vi "Object_Editor_SoftFP.vi"(0 "reference in":refnum<class "Object_Editor.lvclass">, 2 "Floating":bool, 5 "error in (no error)":errorcluster) -> (14 "reference out":refnum<class "Object_Editor.lvclass">, 19 "error out":errorcluster)   [LabVIEW 2022 SP3, in "Object_Editor.lvlib" / "Object_Editor.lvclass"]
uses:
  Object_Editor.lvclass
  <vilib>/picture/picture.llb/imagedata.ctl
  Components/ViPER.lvlibp/ViPER.lvclass
  C:/Projects/Medulla/ViPER/ViPER_ProjectTemplates/ProjectTemplates/Source/Core/ViPER/Components/ViPER.lvlibp/ViPER.lvclass
panel:
  in  "Object Tree":string(tree)
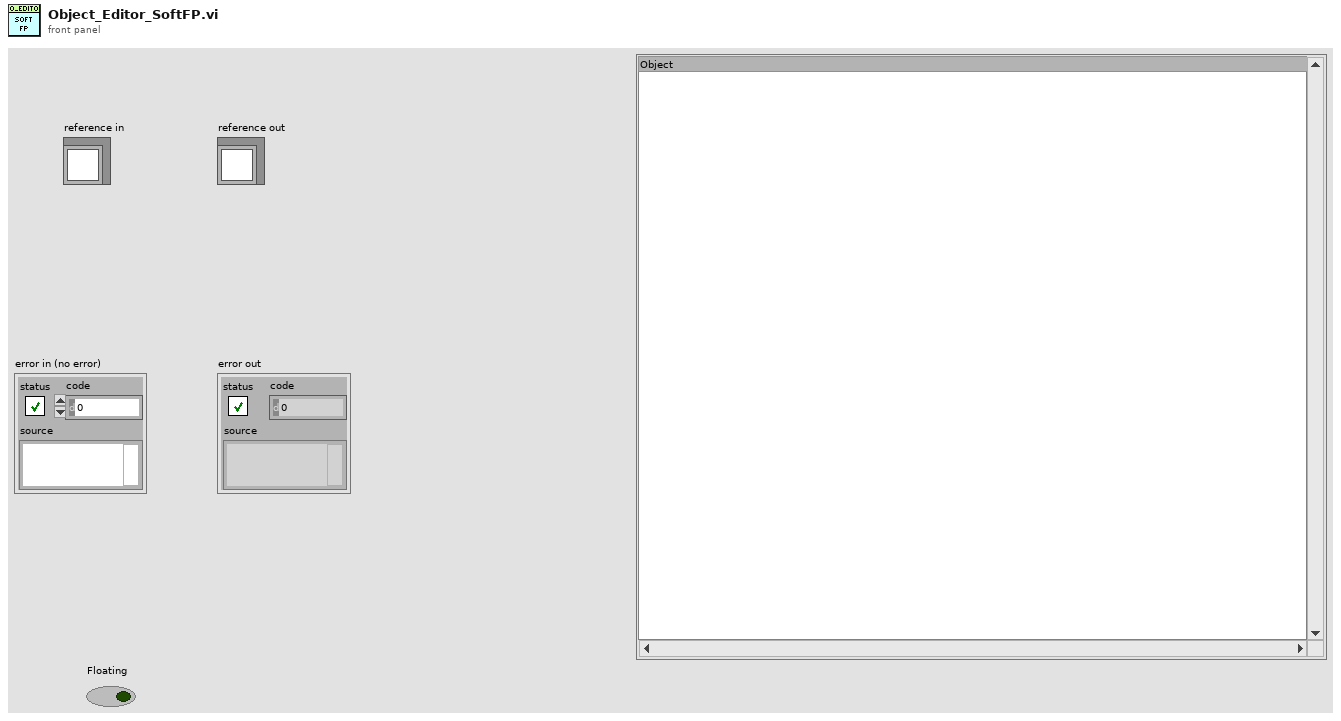
[diagram p1: front panel]
types:
  T1 = enum32{"Invalid", "Standard", "Closed", "Hidden", "Minimized", "Maximized"}
  T2 = typedef "imagedata.ctl" = cluster{"image type":i32, "image depth":i32, "image":u8[], "mask":u8[], "colors":u32[], "Rectangle":cluster{"left":i16, "top":i16, "right":i16, "bottom":i16}}
  T3 = typedef "Object_Editor.lvlib/Object_Editor.lvclass/ObjectAttributes.ctl" = cluster{"Config":T4, "Tree":refnum<vi>, "Mod_Bit":bool, "File_Path":path, "Object":refnum<class "ViPER.lvclass">}
  T4 = typedef "Object_Editor.lvlib/Object_Editor.lvclass/Config.ctl" = cluster{"default":string}
  T5 = typedef "LVPoint32TypeDef.ctl" = cluster{"Horizontal":i32, "Vertical":i32}
  T6 = typedef "Object_Editor.lvlib/Object_Editor.lvclass/TreeItem.ctl" = cluster{"Name":string, "Parent_Tag":string, "Child_Tag":string, "Type":T7, "Data":string}
  T7 = typedef "Object_Editor.lvlib/Object_Editor.lvclass/ItemType.ctl" = enum16{"Object", "Ancestor"}
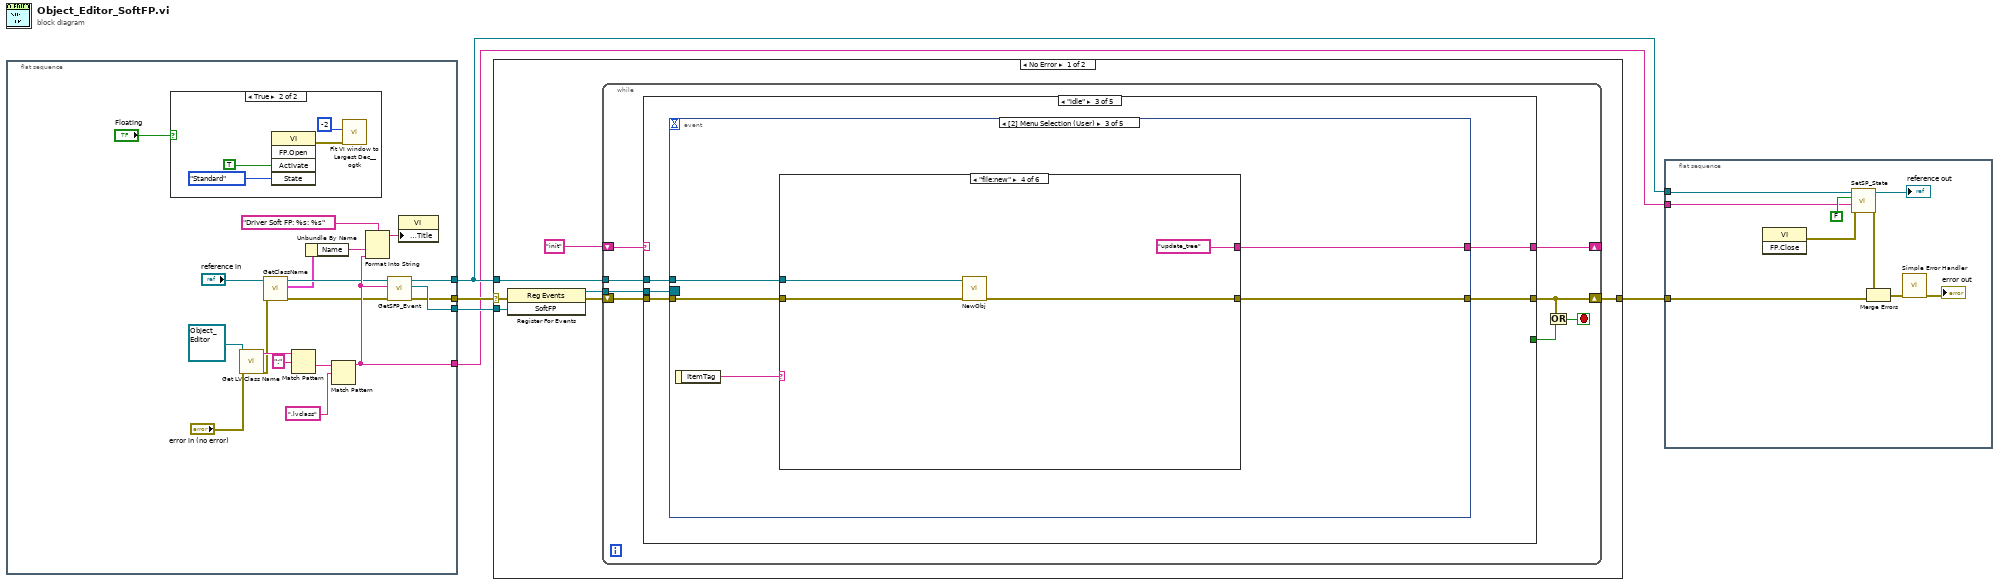
[diagram p0: block diagram]
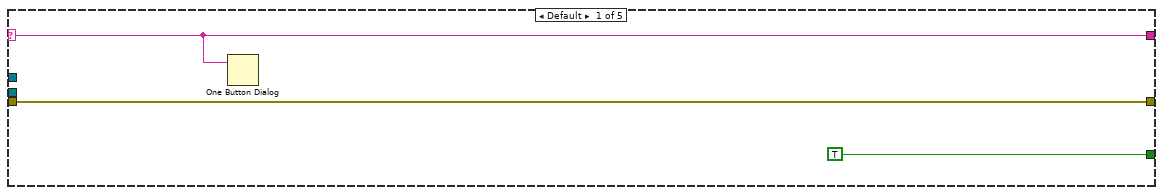
[diagram p3: hidden frame]
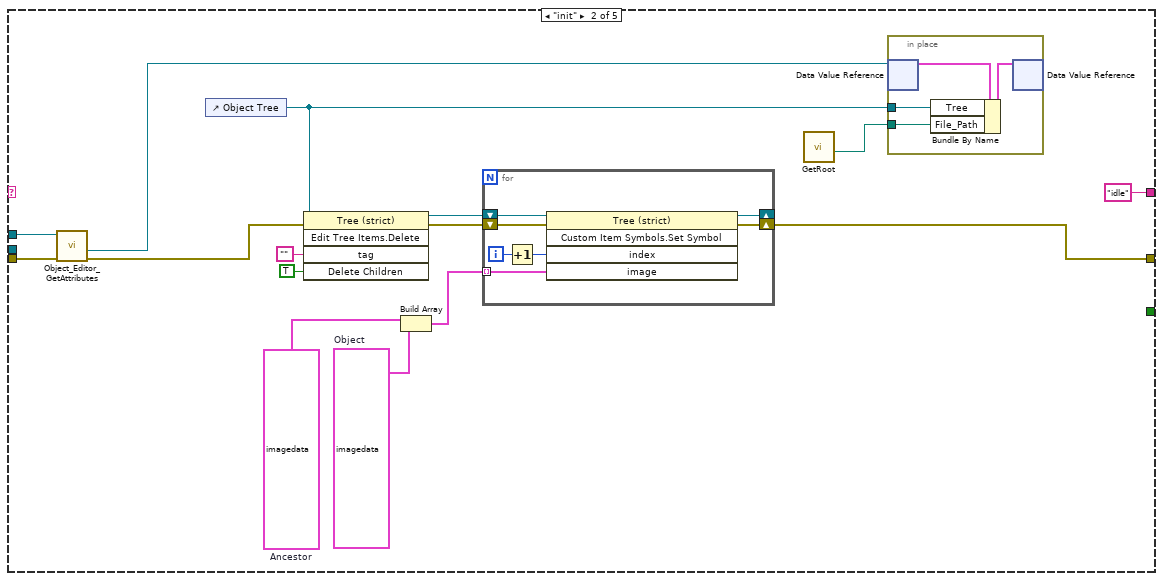
[diagram p4: hidden frame]
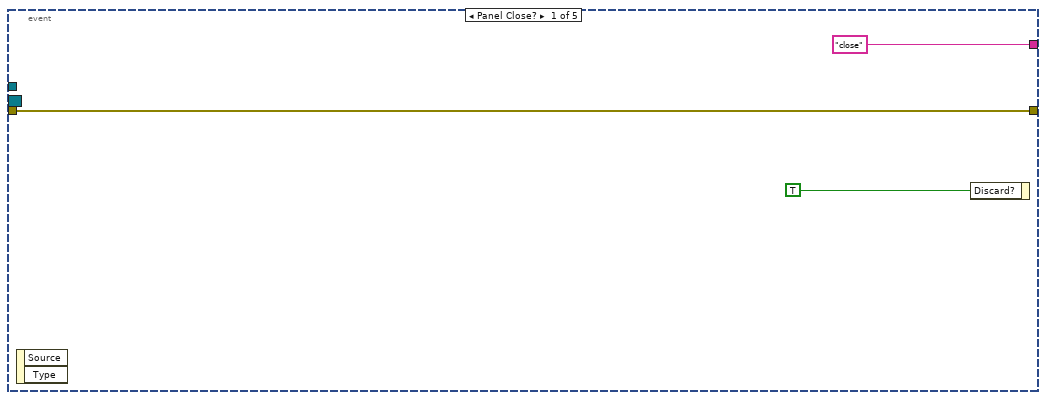
[diagram p5: hidden frame]
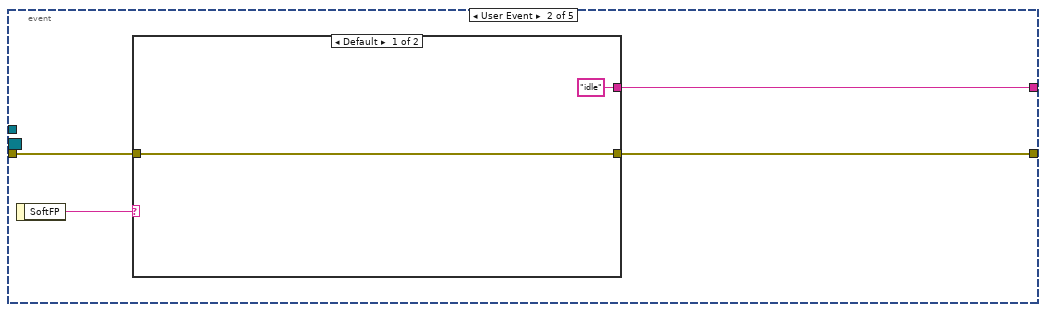
[diagram p6: hidden frame]
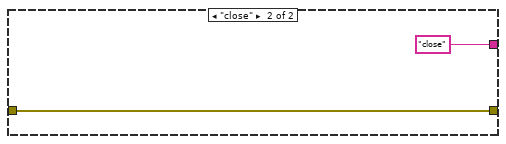
[diagram p7: hidden frame]
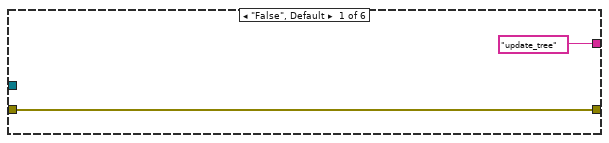
[diagram p8: hidden frame]
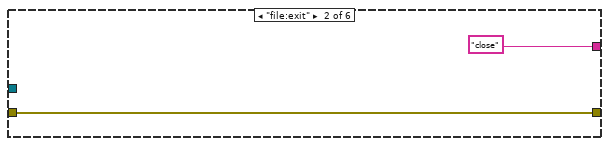
[diagram p9: hidden frame]
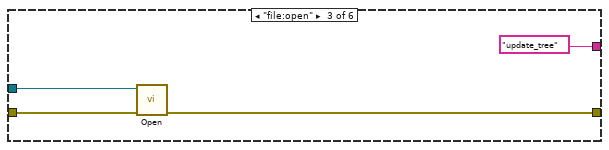
[diagram p10: hidden frame]
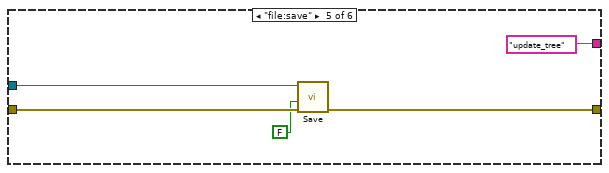
[diagram p11: hidden frame]
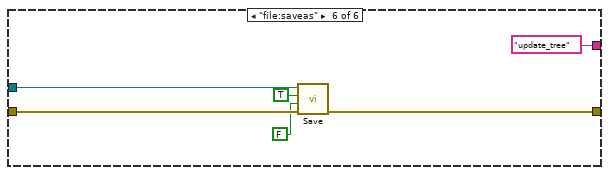
[diagram p12: hidden frame]
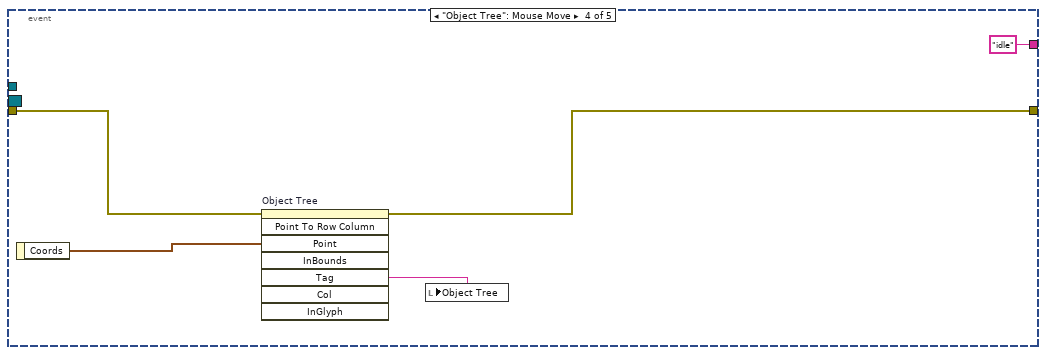
[diagram p13: hidden frame]
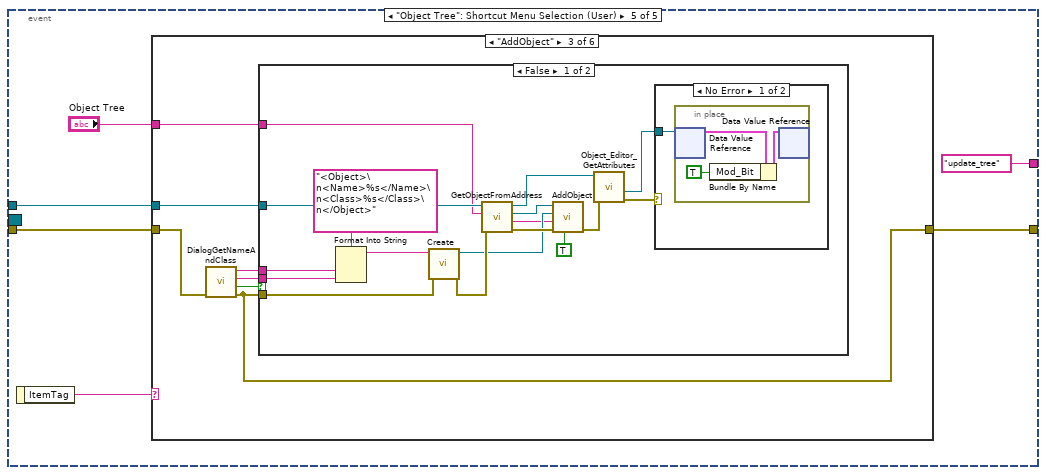
[diagram p14: hidden frame]
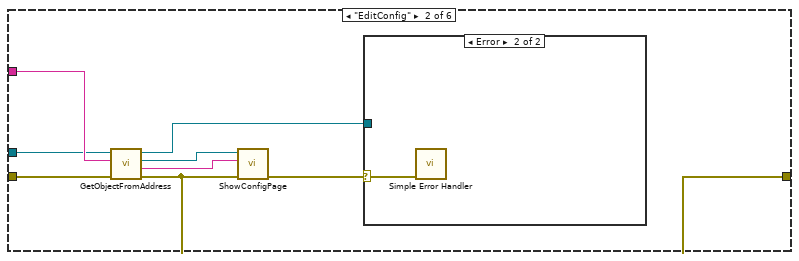
[diagram p16: hidden frame]
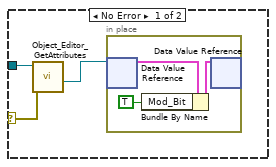
[diagram p17: hidden frame]
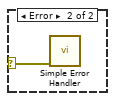
[diagram p18: hidden frame]
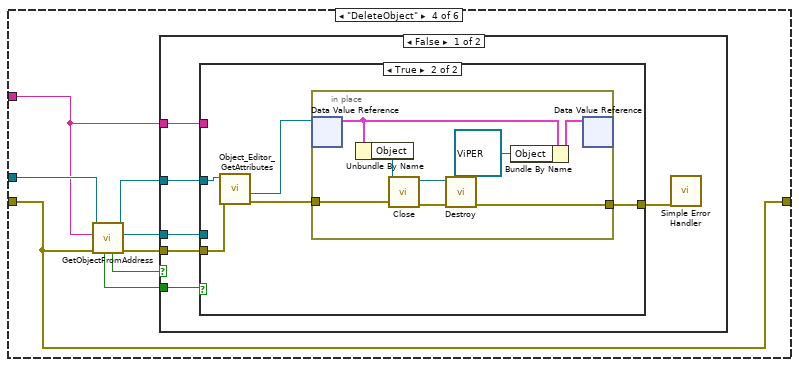
[diagram p20: hidden frame]
diagram:
  n1 = flat-sequence {
    tunnel: [w21] -> w5
    tunnel: [w20] -> w2
    tunnel: [w24] -> w3
    tunnel: [w12] -> w1
    frame #0 {
      n2 = case shown="True" "Floating" {
        frame False {
        }
        frame True {
          n3 = invoke class="VI" method="FP.Open"("Activate"=TRUE ("Activate?"), "State"=T1."Standard") -> (error out=w25:errorcluster)  [unwired: 3 in, 4 out]
          n4 = call <userlib>:"Fit VI window to Largest Dec__ogtk.vi"("error in (no error)"=w25, "border spacing (2 px)"=-2) -> ()  [unwired: 4 in, 2 out]
        }
      }
      n5 = call <vilib>:"Get LV Class Name.vi"("error in (no error)"="error in (no error)", "object"=refnum<class "Object_Editor.lvclass"> refnum ("reference")) -> ("error out"=w11:errorcluster, "class name"=w17:string)  [unwired: 8 in]
      n6 = call "GetClassName.vi"("error in (no error)"=w11, "reference in"="reference in") -> ("error out"=w10:errorcluster, "Details"=w7:cluster{"Name":string, "Class":string}, "reference out"=w8:refnum<class "Object_Editor.lvclass">)  [unwired: 7 in]
      n7 = Match Pattern(string=w17, regular expression=":") -> (after substring=w15:string)  [unwired: 1 in, 3 out]
      n8 = Unbundle By Name(w7) -> ("Name"=w19:string)
      n9 = Match Pattern(string=w15, regular expression=".lvclass") -> (before substring=w12:string)  [unwired: 1 in, 3 out]
      n10 = Format Into String(format string="Driver Soft FP: %s: %s", w19, w12) -> (resulting string=w23:string)  [unwired: 2 in, 1 out]
      n11 = call-dynamic "GetSFP_Event.vi"("error in (no error)"=w10, "Ancestor"=w12, "reference in"=w8) -> ("error out"=w21:errorcluster, "SoftFP"=w24:refnum<user-event>, "reference out"=w20:refnum<class "Object_Editor.lvclass">)  [unwired: 6 in]
      n12 = property class="VI"("Front Panel.Title"=w23) -> ()  [unwired: 2 in, 2 out]
    }
  }
  n13 = case shown="No Error" w5 {
    selector: w5 -> [w33 w306]
    tunnel: [w29 w306] -> w4
    tunnel: w2 -> [w30 _]
    tunnel: w3 -> [w35 _]
    frame No Error {
      n14 = register-events(error in=w33, w35) -> (reference out=w34:refnum<event-registration>, error out=w32:errorcluster)  [unwired: 1 in]
      n15 = while {
        shift-right: [w40] -> w29
        shift-left: w32 -> [w43]
        tunnel: w34 -> [w42]
        tunnel: w30 -> [w41]
        shift-right: [w36] -> _
        shift-left: "init" -> [w37]
        stop <- w39 stop-if-true
        n16 = case shown="\"idle\"" w37 {
          selector: w37 -> [w44 _ _ _ _]
          tunnel: w43 -> [w45 w52 w77 w248 w289]
          tunnel: w42 -> [_ _ w76 _ _]
          tunnel: w41 -> [_ w50 w75 w247 w288]
          tunnel: [w45 w53 w74 w250 w287] -> w40
          tunnel: [TRUE ("Discard?") _ _ _ TRUE ("Discard?")] -> w38
          tunnel: [w44 "idle" w73 "idle" "close"] -> w36
          frame Default {
            n17 = One Button Dialog(message=w44) -> ()  [unwired: 1 in, 1 out]
          }
          frame "init" {
            w56 = T2 {"image type"=0, "image depth"=8, "image"=[0, 0, 0, 0, 0, 2, 16, 28, 17, 7, 0, 0, 0, 0, 0, 0, 0, 0, 0, 1, 15, 27, 35, 35, 35, 33, 18, 8, 0, 0, 0, 0, 0, 0, 14, 26, 35, 35, 35, 35, 35, 35, 35, 35, 21, 11, 0, 0, 4, 20, 35, 35, 35, 35, 35, 35, 35, 35, 35, 35, 35, 35, 19, 5, 9, 31, 24, 30, 35, 35, 35, 35, 35, 35, 35, 35, 29, 25, 32, 10, 9, 34, 34, 31, 24, 30, 35, 35, 35, 35, 29, 25, 32, 36, 36, 10, 9, 34, 34, 34, 34, 31, 24, 30, 29, 25, 32, 36, 36, 36, 36, 10, 9, 34, 34, 34, 34, 34, 34, 31, 32, 36, 36, 36, 36, 36, 36, 10, 9, 34, 34, 34, 34, 34, 34, 34, 36, 36, 36, 36, 36, 36, 36, 10, 9, 34, 34, 34, 34, 34, 34, 34, 36, 36, 36, 36, 36, 36, 36, 10, 9, 34, 34, 34, 34, 34, 34, 34, 36, 36, 36, 36, 36, 36, 36, 10, 9, 34, 34, 34, 34, 34, 34, 34, 36, 36, 36, 36, 36, 36, 36, 10, 3, 22, 34, 34, 34, 34, 34, 34, 36, 36, 36, 36, 36, 36, 23, 6, 0, 0, 12, 22, 34, 34, 34, 34, 36, 36, 36, 36, 23, 13, 0, 0, 0, 0, 0, 0, 12, 22, 34, 34, 36, 36, 23, 13, 0, 0, 0, 0, 0, 0, 0, 0, 0, 0, 12, 22, 23, 13, 0, 0, 0, 0, 0, 0], "mask"=[], "colors"=[16777215, 0, 8421504, 2406046, 3251858, 5592454, 5595526, 4279919, 4279405, 2472602, 5595264, 4278895, 2668443, 5529728, 4409966, 4476268, 4345198, 4410221, 4344685, 4476270, 4346480, 4410478, 2603418, 5595264, 3570304, 4871540, 4476013, 4410221, 4410477, 4410733, 4410989, 2602393, 5529471, 4410477, 2537882, 4410477, 5595264, 0, 0, 0, 0, 0, 0, 0, 0, 0, 0, 0, 0, 0, 0, 0, 0, 0, 0, 0, 0, 0, 0, 0, 0, 0, 0, 0, 0, 0, 0, 0, 0, 0, 0, 0, 0, 0, 0, 0, 0, 0, 0, 0, 0, 0, 0, 0, 0, 0, 0, 0, 0, 0, 0, 0, 0, 0, 0, 0, 0, 0, 0, 0, 0, 0, 0, 0, 0, 0, 0, 0, 0, 0, 0, 0, 0, 0, 0, 0, 0, 0, 0, 0, 0, 0, 0, 0, 0, 0, 0, 0, 0, 0, 0, 0, 0, 0, 0, 0, 0, 0, 0, 0, 0, 0, 0, 0, 0, 0, 0, 0, 0, 0, 0, 0, 0, 0, 0, 0, 0, 0, 0, 0, 0, 0, 0, 0, 0, 0, 0, 0, 0, 0, 0, 0, 0, 0, 0, 0, 0, 0, 0, 0, 0, 0, 0, 0, 0, 0, 0, 0, 0, 0, 0, 0, 0, 0, 0, 0, 0, 0, 0, 0, 0, 0, 0, 0, 0, 0, 0, 0, 0, 0, 0, 0, 0, 0, 0, 0, 0, 0, 0, 0, 0, 0, 0, 0, 0, 0, 0, 0, 0, 0, 0, 0, 0, 0, 0, 0, 0, 0, 0, 0, 0, 0, 0, 0, 0, 0, 0, 0, 0, 0, 0, 0, 0, 0, 0, 0], "Rectangle"={"left"=0, "top"=0, "right"=16, "bottom"=16}}  # Object
            w55 = T2 {"image type"=0, "image depth"=8, "image"=[0, 0, 0, 0, 0, 0, 28, 47, 47, 28, 0, 0, 0, 0, 0, 0, 0, 0, 0, 0, 28, 43, 31, 19, 19, 31, 43, 28, 0, 0, 0, 0, 0, 0, 28, 43, 31, 1, 0, 7, 7, 0, 1, 31, 43, 28, 0, 0, 16, 57, 34, 1, 0, 0, 0, 25, 25, 0, 0, 0, 1, 34, 57, 16, 22, 46, 56, 48, 12, 0, 0, 11, 11, 0, 0, 12, 48, 56, 46, 22, 22, 34, 0, 29, 55, 52, 21, 15, 15, 21, 52, 55, 29, 0, 34, 22, 22, 34, 0, 0, 0, 24, 53, 58, 59, 53, 24, 0, 0, 0, 34, 22, 22, 34, 0, 0, 0, 0, 0, 40, 41, 0, 0, 0, 0, 0, 34, 22, 22, 34, 0, 0, 0, 0, 0, 39, 39, 0, 0, 0, 0, 0, 34, 22, 22, 34, 0, 0, 0, 10, 20, 45, 50, 17, 9, 0, 0, 0, 34, 22, 22, 34, 0, 5, 27, 33, 3, 39, 39, 6, 18, 37, 0, 0, 34, 22, 22, 36, 35, 13, 4, 0, 0, 39, 39, 0, 0, 2, 26, 23, 38, 22, 14, 51, 32, 1, 0, 0, 0, 39, 39, 0, 0, 0, 1, 32, 49, 8, 0, 0, 28, 44, 31, 0, 0, 39, 39, 0, 0, 31, 44, 28, 0, 0, 0, 0, 0, 0, 28, 42, 30, 39, 39, 30, 42, 28, 0, 0, 0, 0, 0, 0, 0, 0, 0, 0, 28, 54, 54, 28, 0, 0, 0, 0, 0, 0], "mask"=[], "colors"=[16777215, 0, 32896, 3394713, 1749913, 2146207, 2865308, 2669716, 4214131, 2406046, 2341271, 2210971, 4216170, 2276249, 3830651, 2603419, 4083052, 2538654, 2669722, 2602902, 2406040, 4475500, 4541040, 2407324, 4475245, 2407323, 2668443, 2603160, 4409966, 4607340, 4344941, 4410732, 4475757, 2472090, 4410222, 2537627, 4152178, 2538138, 3959417, 4476013, 4345198, 4476270, 4410222, 4345197, 4476014, 4023160, 4410477, 4281970, 4410476, 4086643, 3764091, 4086900, 4410733, 4410477, 4410477, 4410477, 4344941, 4344941, 4345967, 4346223, 0, 0, 0, 0, 0, 0, 0, 0, 0, 0, 0, 0, 0, 0, 0, 0, 0, 0, 0, 0, 0, 0, 0, 0, 0, 0, 0, 0, 0, 0, 0, 0, 0, 0, 0, 0, 0, 0, 0, 0, 0, 0, 0, 0, 0, 0, 0, 0, 0, 0, 0, 0, 0, 0, 0, 0, 0, 0, 0, 0, 0, 0, 0, 0, 0, 0, 0, 0, 0, 0, 0, 0, 0, 0, 0, 0, 0, 0, 0, 0, 0, 0, 0, 0, 0, 0, 0, 0, 0, 0, 0, 0, 0, 0, 0, 0, 0, 0, 0, 0, 0, 0, 0, 0, 0, 0, 0, 0, 0, 0, 0, 0, 0, 0, 0, 0, 0, 0, 0, 0, 0, 0, 0, 0, 0, 0, 0, 0, 0, 0, 0, 0, 0, 0, 0, 0, 0, 0, 0, 0, 0, 0, 0, 0, 0, 0, 0, 0, 0, 0, 0, 0, 0, 0, 0, 0, 0, 0, 0, 0, 0, 0, 0, 0, 0, 0, 0, 0, 0, 0, 0, 0, 0, 0, 0, 0, 0, 0, 0, 0, 0, 0, 0, 0, 0, 0, 0, 0, 0, 0, 0, 0, 0, 0, 0, 0], "Rectangle"={"left"=0, "top"=0, "right"=16, "bottom"=16}}  # Ancestor
            n18 = call "Object_Editor_GetAttributes.vi"("error in (no error)"=w52, "reference in"=w50) -> ("error out"=w51:errorcluster, "DataRef"=w49:refnum<data-value>)  [unwired: 6 in, 2 out]
            n19 = control-ref of="Object Tree"() -> (w48:refnum<vi>)
            n20 = invoke class="Tree (strict)" method="Edit Tree Items.Delete"(reference=w48, error in=w51, "tag"="", "Delete Children"=TRUE ("Delete Children?")) -> (reference out=w58:refnum<vi>, error out=w57:errorcluster)  [unwired: 1 in, 3 out]
            n21 = Build Array(w55, w56) -> (w54:T2[])
            n22 = for {
              shift-right: [w71] -> _
              shift-left: w58 -> [w72]
              tunnel: w54 -> [w70] mode=indexing
              shift-right: [w68] -> w53
              shift-left: w57 -> [w69]
              i -> [w67]
              n23 = Increment(x=w67) -> (x+1=w66:i32)
              n24 = invoke class="Tree (strict)" method="Custom Item Symbols.Set Symbol"(reference=w72, error in=w69, "index"=w66, "image"=w70) -> (reference out=w71:refnum<vi>, error out=w68:errorcluster)  [unwired: 1 in, 3 out]
            }
            n25 = call "GetRoot.vi"() -> ("Root"=w47:path)  [unwired: 10 in, 1 out]
            n26 = in-place {
              in-place-border: w48 -> [w63]
              in-place-border: w47 -> [w62]
              n27 = in-place-dvr #1(w49) -> (w65:T3)  [unwired: 1 out]
              n28 = Bundle By Name(cluster=w65, "Tree"=w63, "File_Path"=w62) -> (w64:T3)
              n29 = in-place-dvr #1(w64) -> ()  [unwired: 2 out]
            }
          }
          frame "idle" {
            n30 = event shown="[2] Menu Selection (User)" {
              selector: w76 -> [_ _ _ _ _]
              dyn-events: _ -> [_ _ _ _ _]
              timeout: _ -> [_ _ _ _ _]
              tunnel: w77 -> [w78 w84 w93 w120 w123]
              tunnel: [w78 w82 w91 w119 w122] -> w74
              tunnel: w75 -> [_ _ w92 _ w124]
              tunnel: ["close" w81 w89 "idle" "update_tree"] -> w73
              event Panel Close? {
                n31 = event-data() -> ()  [unwired: 1 in, 2 out]
                n32 = event-data("Discard?"=TRUE) -> ()  [unwired: 1 in, 1 out]
              }
              event User Event {
                n33 = event-data() -> ("SoftFP"=w83:string)  [unwired: 1 in]
                n34 = case shown="Default" w83 {
                  tunnel: w84 -> [w86 w88]
                  tunnel: [w86 w88] -> w82
                  tunnel: ["idle" "close"] -> w81
                  frame Default {
                  }
                  frame "close" {
                  }
                }
              }
              event Menu Selection (User) {
                n35 = event-data() -> ("ItemTag"=w90:string)  [unwired: 1 in]
                n36 = case shown="\"file:new\"" w90 {
                  tunnel: w93 -> [w95 w97 w101 w105 w110 w116]
                  tunnel: w92 -> [_ _ w100 w103 w108 w114]
                  tunnel: [w95 w97 w99 w104 w109 w115] -> w91
                  tunnel: ["update_tree" "close" "update_tree" "update_tree" "update_tree" "update_tree"] -> w89
                  frame "False", Default {
                  }
                  frame "file:exit" {
                  }
                  frame "file:open" {
                    n37 = call "Open.vi"("error in (no error)"=w101, "reference in"=w100) -> ("error out"=w99:errorcluster)  [unwired: 8 in, 1 out]
                  }
                  frame "file:new" {
                    n38 = call "NewObj.vi"("error in (no error)"=w105, "reference in"=w103) -> ("error out"=w104:errorcluster)  [unwired: 8 in, 1 out]
                  }
                  frame "file:save" {
                    n39 = call "Save.vi"("error in (no error)"=w110, "Prompt"=FALSE, "reference in"=w108) -> ("error out"=w109:errorcluster)  [unwired: 7 in, 1 out]
                  }
                  frame "file:saveas" {
                    n40 = call "Save.vi"("error in (no error)"=w116, "Prompt"=FALSE, "Save_As"=TRUE, "reference in"=w114) -> ("error out"=w115:errorcluster)  [unwired: 6 in, 1 out]
                  }
                }
              }
              event "Object Tree": Mouse Move {
                n41 = event-data() -> ("Coords"=w121:T5)  [unwired: 1 in]
                n42 = invoke on="Object Tree" class="Tree (strict)" method="Point To Row Column"(error in=w120, "Point"=w121) -> (error out=w119:errorcluster, "Tag"=w117:string)  [unwired: 6 in, 6 out]
                n43 = local write "Object Tree"(w117) -> ()
              }
              event "Object Tree": Shortcut Menu Selection (User) {
                n44 = event-data() -> ("ItemTag"=w126:string)  [unwired: 1 in]
                n45 = case shown="\"AddObject\"" w126 {
                  tunnel: w123 -> [w128 w134 w149 w175 w228 w240]
                  tunnel: [w128 w132 w144 w175 w218 w235] -> w122
                  tunnel: w124 -> [_ w135 w150 w179 w227 w239]
                  tunnel: "Object Tree" -> [_ w136 w145 w178 w226 w238]
                  frame "False", Default {
                  }
                  frame "EditConfig" {
                    n46 = call "GetObjectFromAddress.vi"("error in (no error)"=w134, "object address"=w136, "reference in"=w135) -> ("error out"=w132:errorcluster, "Ancestor"=w129:string, "object"=w130:refnum<class "ViPER.lvclass">, "reference out"=w133:refnum<class "Object_Editor.lvclass">)  [unwired: 3 in, 2 out]
                    n47 = call-dynamic "ShowConfigPage.vi"("error in (no error)"=w132, "Ancestor"=w129, "Driver in"=w130) -> ("error out"=w131:errorcluster)  [unwired: 7 in, 1 out]
                    n48 = case shown="Error" w131 {
                      selector: w131 -> [w137 w143]
                      tunnel: w133 -> [w139 _]
                      frame No Error {
                        n49 = call "Object_Editor_GetAttributes.vi"("error in (no error)"=w137, "reference in"=w139) -> ("DataRef"=w138:refnum<data-value>)  [unwired: 6 in, 3 out]
                        n50 = in-place {
                          n51 = in-place-dvr #2(w138) -> (w142:T3)  [unwired: 1 out]
                          n52 = Bundle By Name(cluster=w142, "Mod_Bit"=TRUE) -> (w141:T3)
                          n53 = in-place-dvr #2(w141) -> ()  [unwired: 2 out]
                        }
                      }
                      frame Error {
                        n54 = call <vilib>:"Simple Error Handler.vi"("error in (no error)"=w143) -> ()  [unwired: 4 in, 5 out]
                      }
                    }
                  }
                  frame "AddObject" {
                    n55 = call "DialogGetNameAndClass.vi"("error in (no error)"=w149) -> ("error out"=w144:errorcluster, "Cancelled"=w148:bool, "Class"=w147:string, "Name"=w146:string)  [unwired: 7 in]
                    n56 = case shown="False" w148 {
                      tunnel: w150 -> [w167 _]
                      tunnel: w144 -> [w157 _]
                      tunnel: w147 -> [w165 _]
                      tunnel: w146 -> [w164 _]
                      tunnel: w145 -> [w163 _]
                      frame False {
                        n57 = Format Into String(format string="<Object>\n<Name>%s</Name>\n<Class>%s</Class>\n</Object>", w164, w165) -> (resulting string=w155:string)  [unwired: 2 in, 1 out]
                        n58 = call "Create.vi"("error in (no error)"=w157, "Config XML"=w155) -> ("error out"=w156:errorcluster, "reference out"=w154:refnum<class "ViPER.lvclass">)  [unwired: 8 in]
                        n59 = call "GetObjectFromAddress.vi"("error in (no error)"=w156, "object address"=w163, "reference in"=w167) -> ("error out"=w159:errorcluster, "Ancestor"=w153:string, "object"=w158:refnum<class "ViPER.lvclass">, "reference out"=w161:refnum<class "Object_Editor.lvclass">)  [unwired: 3 in, 2 out]
                        n60 = call "AddObject.vi"("donating?"=TRUE, "error in (no error)"=w159, "Ancestor"=w153, "driver"=w154, "reference in"=w158) -> ("error out"=w151:errorcluster)  [unwired: 5 in, 1 out]
                        n61 = call "Object_Editor_GetAttributes.vi"("error in (no error)"=w151, "reference in"=w161) -> ("error out"=w160:errorcluster, "DataRef"=w162:refnum<data-value>)  [unwired: 6 in, 2 out]
                        n62 = case shown="No Error" w160 {
                          selector: w160 -> [_ w172]
                          tunnel: w162 -> [w168 _]
                          frame No Error {
                            n63 = in-place {
                              n64 = in-place-dvr #3(w168) -> (w171:T3)  [unwired: 1 out]
                              n65 = Bundle By Name(cluster=w171, "Mod_Bit"=TRUE) -> (w170:T3)
                              n66 = in-place-dvr #3(w170) -> ()  [unwired: 2 out]
                            }
                          }
                          frame Error {
                            n67 = call <vilib>:"Simple Error Handler.vi"("error in (no error)"=w172) -> ()  [unwired: 4 in, 5 out]
                          }
                        }
                      }
                      frame True {
                      }
                    }
                  }
                  frame "DeleteObject" {
                    n68 = call "GetObjectFromAddress.vi"("error in (no error)"=w175, "object address"=w178, "reference in"=w179) -> ("error out"=w176:errorcluster, "object"=w177:refnum<class "ViPER.lvclass">, "reference out"=w180:refnum<class "Object_Editor.lvclass">, "is ancestor"=w174:bool, "root object"=w173:bool)  [unwired: 3 in, 1 out]
                    n69 = case shown="False" w174 {
                      tunnel: w180 -> [w186 _]
                      tunnel: w178 -> [w185 _]
                      tunnel: w177 -> [w184 _]
                      tunnel: w176 -> [w183 _]
                      tunnel: w173 -> [w182 _]
                      frame False {
                        n70 = case shown="True" w182 {
                          tunnel: w186 -> [w197 w206]
                          tunnel: w185 -> [w196 _]
                          tunnel: w184 -> [w193 _]
                          tunnel: w183 -> [w195 w205]
                          tunnel: [w190 w204] -> w181
                          frame False {
                            w199 = ":" ("delimiter (Tab)")
                            n71 = call <userlib>:"String to 1D Array__ogtk.vi"("delimiter (Tab)"=w199, "string"=w196) -> ("Array of Strings"=w203:string[])  [unwired: 9 in]
                            n72 = Array Size(array=w203) -> (size(s)=w202:i32)
                            n73 = call "GetClassName.vi"("error in (no error)"=w195, "reference in"=w193) -> ("error out"=w194:errorcluster, "Details"=w192:cluster{"Name":string, "Class":string})  [unwired: 7 in, 1 out]
                            n74 = Decrement(x=w202) -> (x-1=w201:i32)
                            n75 = Delete From Array(array=w203, index=w201) -> (array with subset deleted=w200:string[])  [unwired: 1 in, 1 out]
                            n76 = Unbundle By Name(w192) -> ("Name"=w187:string)
                            n77 = call <userlib>:"1D Array to String__ogtk.vi"("delimiter (Tab)"=w199, "Array of Strings"=w200) -> ("delimited string"=w198:string)  [unwired: 9 in]
                            n78 = call "GetObjectFromAddress.vi"("error in (no error)"=w194, "object address"=w198, "reference in"=w197) -> ("error out"=w191:errorcluster, "Ancestor"=w188:string, "object"=w189:refnum<class "ViPER.lvclass">)  [unwired: 3 in, 3 out]
                            n79 = call "RemoveObject.vi"("error in (no error)"=w191, "Ancestor"=w188, "Name"=w187, "reference in"=w189) -> ("error out"=w190:errorcluster)  [unwired: 6 in, 1 out]
                          }
                          frame True {
                            n80 = call "Object_Editor_GetAttributes.vi"("error in (no error)"=w205, "reference in"=w206) -> ("error out"=w208:errorcluster, "DataRef"=w207:refnum<data-value>)  [unwired: 6 in, 2 out]
                            n81 = in-place {
                              in-place-border: w208 -> [w213]
                              in-place-border: [w210] -> w204
                              n82 = in-place-dvr #4(w207) -> (w216:T3)  [unwired: 1 out]
                              n83 = Unbundle By Name(w216) -> ("Object"=w214:refnum<class "ViPER.lvclass">)
                              n84 = call-dynamic "Close.vi"("error in (no error)"=w213, "reference in"=w214) -> ("error out"=w212:errorcluster, "reference out"=w211:refnum<class "ViPER.lvclass">)  [unwired: 8 in]
                              n85 = call "Destroy.vi"("error in (no error)"=w212, "reference in"=w211) -> ("error out"=w210:errorcluster)  [unwired: 9 in]
                              n86 = Bundle By Name(cluster=w216, "Object"=refnum<class "ViPER.lvclass"> refnum) -> (w215:T3)
                              n87 = in-place-dvr #4(w215) -> ()  [unwired: 2 out]
                            }
                          }
                        }
                        n88 = call <vilib>:"Simple Error Handler.vi"("error in (no error)"=w181) -> ()  [unwired: 4 in, 5 out]
                      }
                      frame True {
                      }
                    }
                  }
                  frame "ShowSFP" {
                    n89 = call "GetObjectFromAddress.vi"("error in (no error)"=w228, "object address"=w226, "reference in"=w227) -> ("error out"=w218:errorcluster, "Ancestor"=w225:string, "object"=w221:refnum<class "ViPER.lvclass">)  [unwired: 3 in, 3 out]
                    n90 = call "GetInitOK.vi"("error in (no error)"=w218, "reference in"=w221) -> ("error out"=w217:errorcluster, "init_ok"=w219:bool, "reference out"=w220:refnum<class "ViPER.lvclass">)  [unwired: 7 in]
                    n91 = case shown="False" w219 {
                      tunnel: w217 -> [w232 w234]
                      tunnel: w220 -> [w230 w233]
                      tunnel: [w231 w234] -> w224
                      tunnel: [w229 w233] -> w223
                      frame False {
                        n92 = call-dynamic "Init.vi"("error in (no error)"=w232, "reference in"=w230) -> ("error out"=w231:errorcluster, "reference out"=w229:refnum<class "ViPER.lvclass">)  [unwired: 8 in]
                      }
                      frame True {
                      }
                    }
                    n93 = call-dynamic "ShowSoftPanel.vi"("error in (no error)"=w224, "Ancestor"=w225, "Driver in"=w223) -> ("error out"=w222:errorcluster)  [unwired: 6 in, 2 out]
                    n94 = call <vilib>:"Simple Error Handler.vi"("error in (no error)"=w222) -> ()  [unwired: 4 in, 5 out]
                  }
                  frame "InitObject" {
                    n95 = call "GetObjectFromAddress.vi"("error in (no error)"=w240, "object address"=w238, "reference in"=w239) -> ("error out"=w235:errorcluster, "object"=w237:refnum<class "ViPER.lvclass">)  [unwired: 3 in, 4 out]
                    n96 = call-dynamic "Init.vi"("error in (no error)"=w235, "reference in"=w237) -> ("error out"=w236:errorcluster)  [unwired: 8 in, 1 out]
                    n97 = call <vilib>:"Simple Error Handler.vi"("error in (no error)"=w236) -> ()  [unwired: 4 in, 5 out]
                  }
                }
              }
            }
          }
          frame "update_tree" {
            # "Want the class name in the 2nd column"
            n98 = call "Object_Editor_GetAttributes.vi"("error in (no error)"=w248, "reference in"=w247) -> ("error out"=w244:errorcluster, "Data"=w246:T3)  [unwired: 6 in, 2 out]
            n99 = Unbundle By Name(w246) -> ("Tree"=w245:refnum<vi>, "Object"=w242:refnum<class "ViPER.lvclass">)
            n100 = call "GetClassName.vi"("error in (no error)"=w244, "reference in"=w242) -> ("error out"=w243:errorcluster, "reference out"=w241:refnum<class "ViPER.lvclass">)  [unwired: 7 in, 1 out]
            n101 = case shown="No Error" w243 {
              tunnel: [w255 w282] -> w250
              tunnel: w245 -> [w253 w281]
              tunnel: w241 -> [w252 _]
              tunnel: w244 -> [w251 w282]
              frame No Error {
                w258 = ""
                n102 = call-dynamic "SerializeObject.vi"("error in (no error)"=w251, "ViPER_Base in"=w252) -> ("error out"=w262:errorcluster, "Object XML"=w261:string)  [unwired: 7 in, 1 out]
                n103 = call "ParseObject.vi"("error in (no error)"=w262, "Tag In"=w258, "Object_XML"=w261) -> ("error out"=w259:errorcluster, "Array"=w254:T6[])  [unwired: 7 in]
                n104 = invoke class="Tree (strict)" method="Edit Tree Items.Delete"(reference=w253, error in=w259, "tag"=w258, "Delete Children"=TRUE ("Delete Children?")) -> (reference out=w257:refnum<vi>, error out=w256:errorcluster)  [unwired: 1 in, 3 out]
                n105 = for {
                  tunnel: w257 -> [w273]
                  tunnel: w254 -> [w276] mode=indexing
                  shift-right: [w269] -> w255
                  shift-left: w256 -> [w271]
                  n106 = Unbundle By Name(w276) -> ("Parent_Tag"=w275:string, "Name"=w274:string, "Child_Tag"=w268:string, "Type"=w264:T7)
                  n107 = invoke class="Tree (strict)" method="Edit Tree Items.Add Item"(reference=w273, error in=w271, "Parent Tag"=w275, "Child Position"=-1, "Left Cell"=w274, "Child Tag"=w268, "Child Only?"=FALSE) -> (reference out=w272:refnum<vi>, error out=w270:errorcluster, "Edit Tree Items:Add Item"=w267:string)  [unwired: 2 in, 6 out]
                  n108 = case shown="\"Ancestor\"" w264 {
                    tunnel: [2 ("Active Item:Symbol Index") 1 ("Active Item:Symbol Index")] -> w263
                    frame "Object", Default {
                    }
                    frame "Ancestor" {
                    }
                  }
                  n109 = property class="Tree (strict)"(reference=w272, error in=w270, "Active Item Tag"=w267, "Glyph"=w263) -> (error out=w269:errorcluster)  [unwired: 1 out]
                }
              }
              frame Error {
                n110 = invoke class="Tree (strict)" method="Edit Tree Items.Delete"(reference=w281, "tag"="", "Delete Children"=TRUE ("Delete Children?")) -> ()  [unwired: 2 in, 5 out]
              }
            }
          }
          frame "close" {
            n111 = call "Object_Editor_GetAttributes.vi"("error in (no error)"=w289, "reference in"=w288) -> ("error out"=w293:errorcluster, "Data"=w292:T3, "reference out"=w290:refnum<class "Object_Editor.lvclass">)  [unwired: 6 in, 1 out]
            n112 = Unbundle By Name(w292) -> ("Object"=w284:refnum<class "ViPER.lvclass">, "Mod_Bit"=w291:bool)
            n113 = case shown="True" w291 {
              tunnel: w293 -> [w302 w305]
              tunnel: [w302 w304] -> w286
              tunnel: w290 -> [_ w303]
              frame False {
              }
              frame True {
                n114 = call "Save.vi"("error in (no error)"=w305, "reference in"=w303) -> ("error out"=w304:errorcluster)  [unwired: 8 in, 1 out]
              }
            }
            n115 = call "GetInitOK.vi"("error in (no error)"=w286, "reference in"=w284) -> ("error out"=w285:errorcluster, "reference out"=w283:refnum<class "ViPER.lvclass">)  [unwired: 7 in, 1 out]
            n116 = case shown="No Error" w285 {
              tunnel: [w297 w301] -> w287
              tunnel: w286 -> [w300 w301]
              tunnel: w283 -> [w299 _]
              frame No Error {
                n117 = call-dynamic "Close.vi"("error in (no error)"=w300, "reference in"=w299) -> ("error out"=w298:errorcluster, "reference out"=w296:refnum<class "ViPER.lvclass">)  [unwired: 8 in]
                n118 = call "Destroy.vi"("error in (no error)"=w298, "reference in"=w296) -> ("error out"=w297:errorcluster)  [unwired: 9 in]
              }
              frame Error {
              }
            }
          }
        }
        n119 = Or(x=w40, y=w38) -> (x .or. y?=w39:bool)
      }
    }
    frame Error {
    }
  }
  n120 = flat-sequence {
    tunnel: w4 -> [w313]
    tunnel: w2 -> [w310]
    tunnel: w1 -> [w307]
    frame #0 {
      n121 = invoke class="VI" method="FP.Close"() -> (error out=w312:errorcluster)  [unwired: 3 in, 2 out]
      n122 = call "SetSP_State.vi"("error in (no error)"=w312, "Ancestor"=w307, "SP Open"=FALSE, "reference in"=w310) -> ("error out"=w311:errorcluster, "reference out"=→"reference out":refnum<class "Object_Editor.lvclass">)  [unwired: 6 in]
      n123 = Merge Errors(w311, w313) -> (w315:errorcluster)
      n124 = call <vilib>:"Simple Error Handler.vi"("error in (no error)"=w315) -> ("error out"=→"error out":errorcluster)  [unwired: 4 in, 4 out]
    }
  }
